vi "sub_XY Amplitude Regular.vi"(10 "Y Amplitude":dbl, 11 "X Amplitude":dbl) -> (2 "Y Amplitude Out":fxp<+,16,0> format="%.16g", 3 "X Amplitude Out":fxp<+,16,0> format="%.16g")   [LabVIEW 2015]
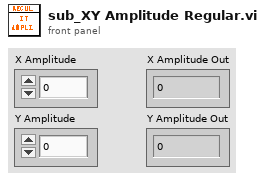
[diagram p1: front panel]
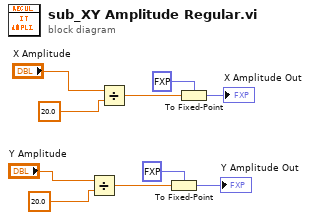
[diagram p0: block diagram]
diagram:
  n1 = Divide(x="Y Amplitude", y=20.0) -> (x/y=w9:dbl)
  n2 = Divide(x="X Amplitude", y=20.0) -> (x/y=w6:dbl)
  n3 = To Fixed-Point(fixed-point type=fxp<+,16,0> 0.0 ("Y Amplitude"), number=w9) -> (fixed-point=→"Y Amplitude Out":fxp<+,16,0>)
  n4 = To Fixed-Point(fixed-point type=fxp<+,16,0> 0.0 ("Y Amplitude"), number=w6) -> (fixed-point=→"X Amplitude Out":fxp<+,16,0>)
